vi "Read Measurements.vi"(8 "error in":errorcluster, 9 "Data Frame Format In":T1, 10 "Unit ID (A)":string="A", 11 "VISA Session In":refnum<visa-resource-name>="Alicat") -> (0 "error out":errorcluster, 1 "Data Frame Format Out":T1, 2 "Data Cluster":T2, 3 "VISA Session Out":refnum<visa-resource-name>, 4 "Unknown Dataframe Info":bool, 5 "Error/Overrange/Unknown String":string, 6 "Error Present":bool, 7 "Range Exceeded":bool)   [LabVIEW 2024]
doc: "Polls the Alicat device for its data frame and outputs cluster of data, retrieved/used data flags, and error/overrange/unknown indicators and strings. Data is parsed according to data flag inputs, and if none are present the device will query the data flags (adding a considerable amount of time to the VI's execution)."
uses:
  <vilib>/Instr/_visa.llb/VISA Flush IO Buffer Mask.ctl
panel:
  # "Totalizer Timer"
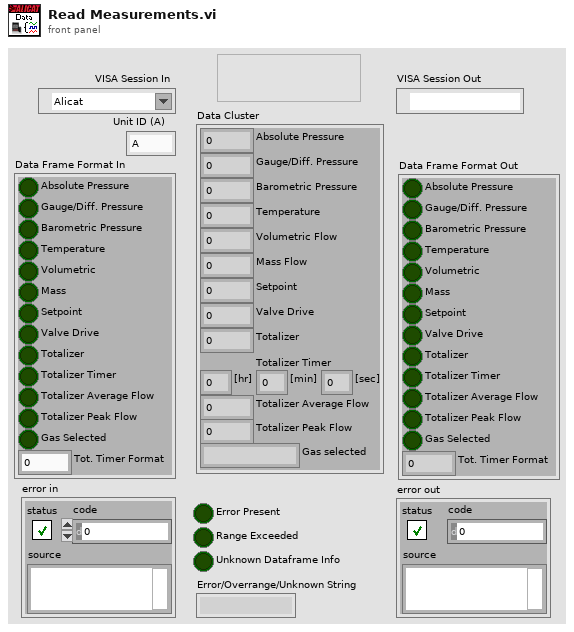
[diagram p1: front panel]
types:
  T1 = cluster{"Absolute Pressure":bool, "Gauge/Diff. Pressure":bool, "Barometric Pressure":bool, "Temperature":bool, "Volumetric":bool, "Mass":bool, "Setpoint":bool, "Valve Drive":bool, "Totalizer":bool, "Totalizer Timer":bool, "Totalizer Average Flow":bool, "Totalizer Peak Flow":bool, "Gas Selected":bool, "Tot. Timer Format":u16}
  T2 = cluster{"Absolute Pressure":dbl, "Gauge/Diff. Pressure":dbl, "Barometric Pressure":dbl, "Temperature":dbl, "Volumetric Flow":dbl, "Mass Flow":dbl, "Setpoint":dbl, "Valve Drive":dbl, "Totalizer":dbl, "[hr]":dbl, "[min]":dbl, "[sec]":dbl, "Totalizer Average Flow":dbl, "Totalizer Peak Flow":dbl, "Gas selected":string}
  T3 = cluster{"Absolute Pressure":dbl, "Gauge/Diff. Pressure":dbl, "Barometric Pressure":dbl, "Temperature":dbl, "Volumetric":dbl, "Mass":dbl, "Setpoint":dbl, "Valve Drive":dbl, "Totalizer":dbl, "[hr]":dbl, "[min]":dbl, "[sec]":dbl, "Totalizer Average Flow":dbl, "Totalizer Peak Flow":dbl, "Gas selected":string}
  T4 = typedef "VISA Flush IO Buffer Mask.ctl" = u16
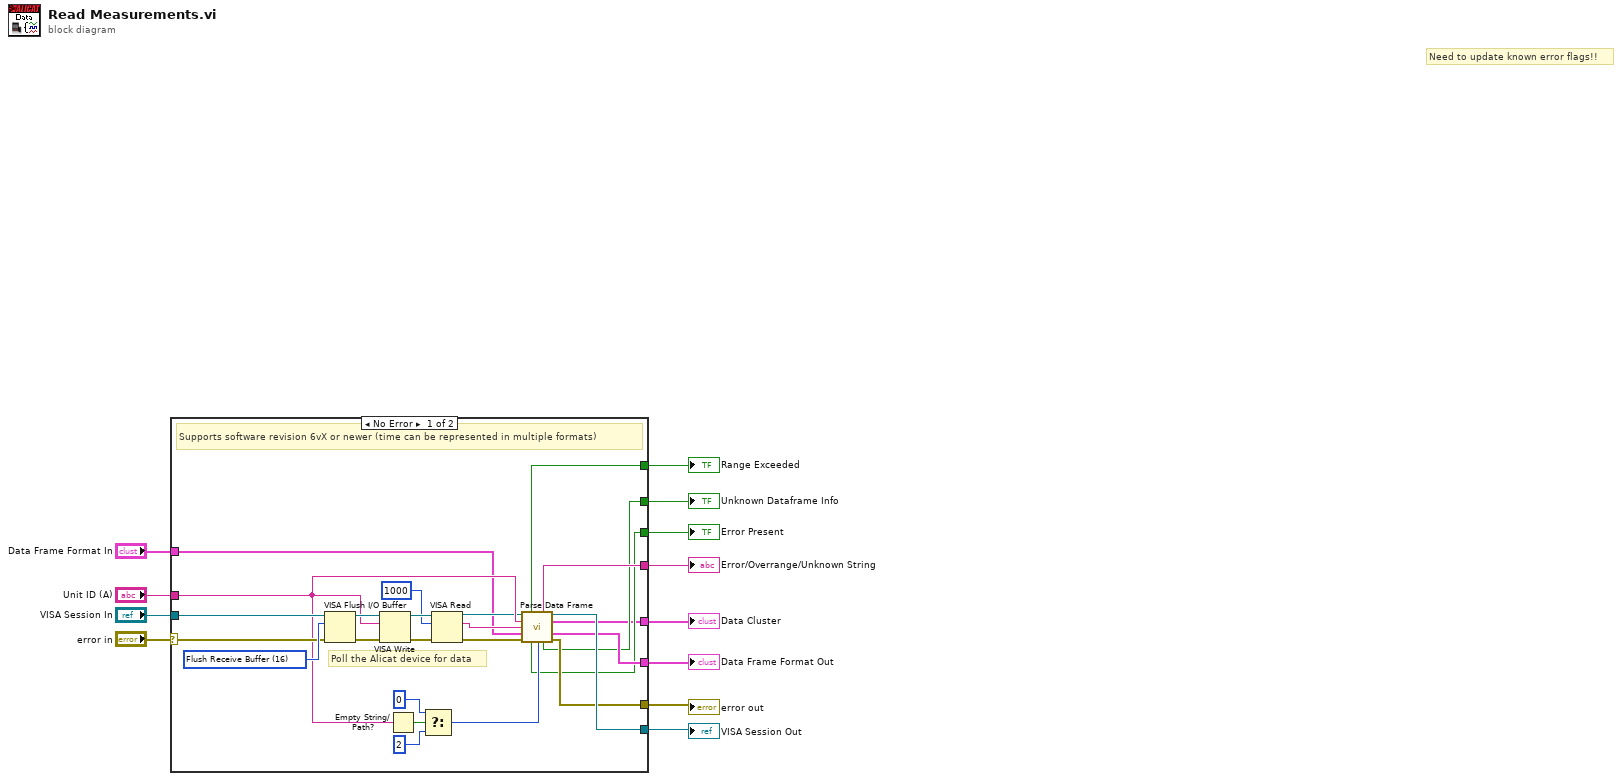
[diagram p0: block diagram]
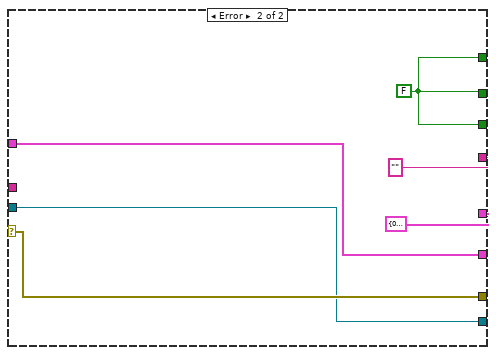
[diagram p2: hidden frame]
diagram:
  # "Need to update known error flags!!"
  n1 = case shown="No Error" "error in" {
    selector: "error in" -> [w26 w43]
    tunnel: "VISA Session In" -> [w25 w42]
    tunnel: "Unit ID (A)" -> [w24 _]
    tunnel: [w14 w39] -> w11
    tunnel: [w20 w39] -> w10
    tunnel: [w15 w39] -> w9
    tunnel: [w19 ""] -> w8
    tunnel: [w18 w42] -> w7
    tunnel: [w17 w43] -> w6
    tunnel: "Data Frame Format In" -> [w21 w41]
    tunnel: [w16 w41] -> w2
    tunnel: [w13 T3 {"Absolute Pressure"=0.0, "Gauge/Diff. Pressure"=0.0, "Barometric Pressure"=0.0, "Temperature"=0.0, "Volumetric"=0.0, "Mass"=0.0, "Setpoint"=0.0, "Valve Drive"=0.0, "Totalizer"=0.0, "[hr]"=0.0, "[min]"=0.0, "[sec]"=0.0, "Totalizer Average Flow"=0.0, "Totalizer Peak Flow"=0.0, "Gas selected"=""} ("Data Cluster 2")] -> w5
    frame No Error {
      w32 = T4 16 items=["Flush Receive Buffer"=16, "Write Transmit Buffer to Device"=32, "Flush Receive Buffer (No I/O)"=64, "Flush Transmit Buffer"=128] ("Mask")
      # "Poll the Alicat device for data"
      # "Supports software revision 6vX or newer (time can be represented in multiple formats)"
      n2 = VISA Flush I/O Buffer(VISA resource name=w25, mask (16)=w32, error in (no error)=w26) -> (VISA resource name out=w30:refnum<visa-resource-name>, error out=w28:errorcluster)
      n3 = VISA Write(VISA resource name=w30, write buffer=w24, error in (no error)=w28) -> (VISA resource name out=w31:refnum<visa-resource-name>, error out=w29:errorcluster)  [unwired: 1 out]
      n4 = Empty String/Path?(string/path=w24) -> (empty?=w33:bool)
      n5 = Select(t=u32 0, s=w33, f=u32 2) -> (s? t:f=w36:u32)
      n6 = VISA Read(VISA resource name=w31, byte count=u32 1000, error in (no error)=w29) -> (VISA resource name out=w22:refnum<visa-resource-name>, read buffer=w37:string, error out=w23:errorcluster)  [unwired: 1 out]
      n7 = call "Parse Data Frame.vi"("VISA Session In"=w22, "Unit ID (A)"=w24, "Data Frame Input"=w37, "Data Frame Format In"=w21, "error in"=w23, "Offset (2 if polling, 0 if streaming)"=w36) -> ("Range Exceeded"=w20:bool, "Error/Overrange/Unknown String"=w19:string, "VISA Session Out"=w18:refnum<visa-resource-name>, "Data Cluster"=w13:T2, "Data Frame Format Out"=w16:T1, "Error Present"=w14:bool, "Unknown Dataframe Info"=w15:bool, "error out"=w17:errorcluster)  [unwired: 2 in]
    }
    frame Error {
      w39 = FALSE
    }
  }
  "error out" <- w6
  "VISA Session Out" <- w7
  "Error Present" <- w11
  "Range Exceeded" <- w10
  "Unknown Dataframe Info" <- w9
  "Error/Overrange/Unknown String" <- w8
  "Data Cluster" <- w5
  "Data Frame Format Out" <- w2
